vi "Get Updated Center of Mass.vi"(10 "Current traced points [pix]":cluster{"X":dbl, "Y":dbl}[](array[cluster]), 11 "Objects Description[pix]":T1(array[cluster])) -> (2 "Objects index":i32[](array[numeric]), 3 "Traced Object [pix]":T1(array[cluster]))   [LabVIEW 2012, in "Visual Analyser.lvlib"]
uses:
  Visual Analyser.lvlib
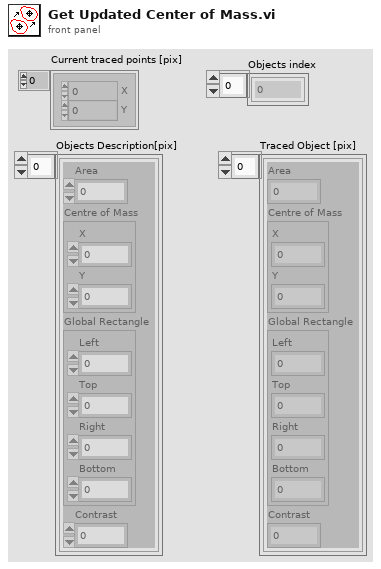
[diagram p1: front panel]
types:
  T1 = cluster{"Area":dbl, "Centre of Mass":cluster{"X":dbl, "Y":dbl}, "Global Rectangle":cluster{"Left":dbl, "Top":dbl, "Right":dbl, "Bottom":dbl}, "Contrast":dbl}[]
  T2 = cluster{"Left":dbl, "Top":dbl, "Right":dbl, "Bottom":dbl}
  T3 = cluster{"Area":dbl, "Centre of Mass":cluster{"X":dbl, "Y":dbl}, "Global Rectangle":cluster{"Left":dbl, "Top":dbl, "Right":dbl, "Bottom":dbl}, "Contrast":dbl}
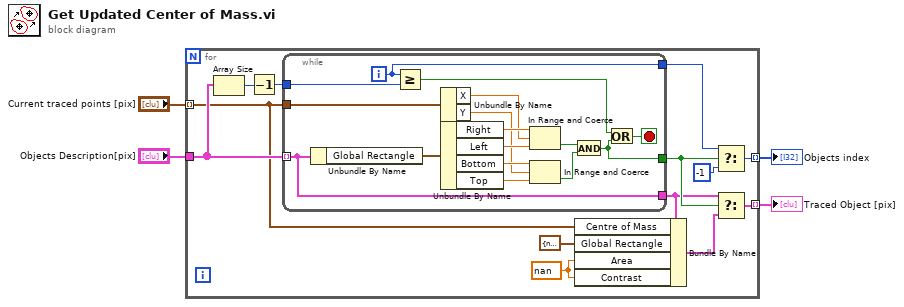
[diagram p0: block diagram]
diagram:
  n1 = for {
    tunnel: "Objects Description[pix]" -> [w12]
    tunnel: "Current traced points [pix]" -> [w7] mode=indexing
    tunnel: [w15] -> w3 mode=indexing
    tunnel: [w13] -> w1 mode=indexing
    w5 = nan ("Area")
    n2 = Array Size(array=w12) -> (size(s)=w17:i32)
    n3 = Decrement(x=w17) -> (x-1=w16:i32)
    n4 = while {
      tunnel: w12 -> [w19] mode=indexing
      tunnel: w7 -> [w18]
      tunnel: w16 -> [w24]
      tunnel: [w22] -> w14
      tunnel: [w20] -> w11
      tunnel: [w19] -> w9
      i -> [w20]
      stop <- w23 stop-if-true
      n5 = Unbundle By Name(w19) -> ("Global Rectangle"=w21:T2)
      n6 = Greater Or Equal?(x=w20, y=w24) -> (x >= y?=w25:bool)
      n7 = Unbundle By Name(w18) -> ("X"=w29:dbl, "Y"=w28:dbl)
      n8 = Unbundle By Name(w21) -> ("Right"=w33:dbl, "Left"=w32:dbl, "Bottom"=w31:dbl, "Top"=w30:dbl)
      n9 = In Range and Coerce(upper limit=w33, x=w29, lower limit=w32) -> (In Range?=w27:bool)  [unwired: 1 out]
      n10 = In Range and Coerce(upper limit=w31, x=w28, lower limit=w30) -> (In Range?=w26:bool)  [unwired: 1 out]
      n11 = And(x=w27, y=w26) -> (x .and. y?=w22:bool)
      n12 = Or(x=w25, y=w22) -> (x .or. y?=w23:bool)
    }
    n13 = Bundle By Name(cluster=w9, "Centre of Mass"=w7, "Global Rectangle"=T2 {"Left"=nan, "Top"=nan, "Right"=nan, "Bottom"=nan}, "Area"=w5, "Contrast"=w5) -> (w8:T3)
    n14 = Select(t=w11, s=w14, f=-1) -> (s? t:f=w15:i32)
    n15 = Select(t=w9, s=w14, f=w8) -> (s? t:f=w13:T3)
  }
  "Objects index" <- w3
  "Traced Object [pix]" <- w1
